vi "WPI_CameraPublish Settings.vi"(8 "Name":string, 9 "Table":string, 11 "CameraDevRef":T1) -> ()   [LabVIEW 2017]
uses:
  <vilib>/Rock Robotics/WPI/Camera/WPI_CameraDevRef.ctl
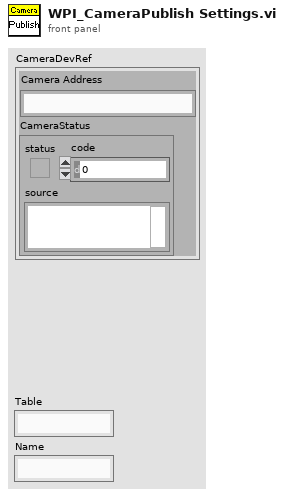
[diagram p1: front panel]
types:
  T1 = typedef "WPI_CameraDevRef.ctl" = cluster{"Camera Address":string, "CameraStatus":errorcluster}
  T2 = typedef "WPI_CameraImageSize.ctl" = enum16{"640x480", "320x240", "160x120", "Custom"}
  T3 = typedef "WPI_CameraFrameRate.ctl" = u32
  T4 = typedef "WPI_CameraExposure Values.ctl" = enum16{"Auto", "Flicker-free 50 Hz", "Flicker-free 60 Hz", "Hold current", "Custom"}
  T5 = typedef "WPI_CameraWhite Balance Values.ctl" = enum16{"Auto", "Fixed indoor", "Fixed outdoor 1", "Fixed outdoor 2", "Fixed fluorescent 1", "Fixed fluorescent 2", "Hold current", "Custom"}
  T6 = typedef "WPI_CameraExposure Priority Values.ctl" = enum16{"None", "Prioritize frame rate", "Prioritize image quality"}
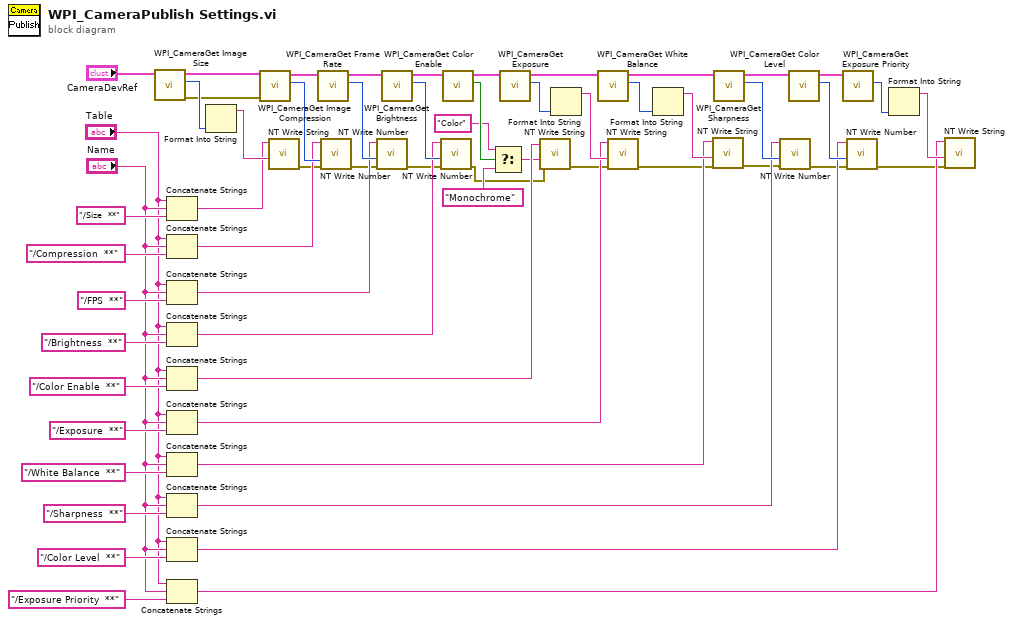
[diagram p0: block diagram]
diagram:
  n1 = call <vilib>:"WPI_CameraGet Image Size.vi"("CameraDevRef"="CameraDevRef") -> ("error out"=w10:errorcluster, "Image Size"=w58:T2, "CameraDevRef Out"=w54:T1)  [unwired: 7 in, 1 out]
  n2 = Concatenate Strings("Table", "Name", "/Size  **") -> (w49:string)
  n3 = Concatenate Strings("Table", "Name", "/Compression  **") -> (w48:string)
  n4 = Concatenate Strings("Table", "Name", "/FPS  **") -> (w47:string)
  n5 = Concatenate Strings("Table", "Name", "/Brightness  **") -> (w43:string)
  n6 = Concatenate Strings("Table", "Name", "/Color Enable  **") -> (w15:string)
  n7 = Concatenate Strings("Table", "Name", "/Exposure  **") -> (w32:string)
  n8 = Concatenate Strings("Table", "Name", "/White Balance  **") -> (w31:string)
  n9 = Concatenate Strings("Table", "Name", "/Sharpness  **") -> (w19:string)
  n10 = Concatenate Strings("Table", "Name", "/Color Level  **") -> (w18:string)
  n11 = Concatenate Strings("Table", "Name", "/Exposure Priority  **") -> (w17:string)
  n12 = Format Into String(w58) -> (resulting string=w59:string)  [unwired: 3 in, 1 out]
  n13 = call <vilib>:"WPI_CameraGet Image Compression.vi"("error in (no error)"=w10, "CameraDevRef"=w54) -> ("Compression"=w55:i32, "CameraDevRef Out"=w57:T1)  [unwired: 7 in, 1 out]
  n14 = call <vilib>:"NT Write String.vi"("String"=w59, "Name"=w49) -> ("error out"=w9:errorcluster)  [unwired: 9 in]
  n15 = call <vilib>:"WPI_CameraGet Frame Rate.vi"("CameraDevRef"=w57) -> ("Frame Rate (fps)"=w56:T3, "CameraDevRef Out"=w46:T1)  [unwired: 8 in, 1 out]
  n16 = call <vilib>:"NT Write Number.vi"("error in"=w9, "Numeric"=w55, "Name"=w48) -> ("error out"=w8:errorcluster)  [unwired: 8 in]
  n17 = call <vilib>:"NT Write Number.vi"("error in"=w8, "Numeric"=w56, "Name"=w47) -> ("error out"=w7:errorcluster)  [unwired: 8 in]
  n18 = call <vilib>:"WPI_CameraGet Brightness.vi"("CameraDevRef"=w46) -> ("Brightness"=w45:i32, "CameraDevRef Out"=w42:T1)  [unwired: 8 in, 1 out]
  n19 = call <vilib>:"NT Write Number.vi"("error in"=w7, "Numeric"=w45, "Name"=w43) -> ("error out"=w6:errorcluster)  [unwired: 8 in]
  n20 = call <vilib>:"WPI_CameraGet Color Enable.vi"("CameraDevRef"=w42) -> ("Color Enabled"=w13:bool, "CameraDevRef Out"=w41:T1)  [unwired: 8 in, 1 out]
  n21 = Select(t="Color", s=w13, f="Monochrome") -> (s? t:f=w14:string)
  n22 = call <vilib>:"WPI_CameraGet Exposure.vi"("CameraDevRef"=w41) -> ("Exposure"=w37:T4, "CameraDevRef Out"=w40:T1)  [unwired: 7 in, 2 out]
  n23 = call <vilib>:"NT Write String.vi"("error in"=w6, "String"=w14, "Name"=w15) -> ("error out"=w5:errorcluster)  [unwired: 8 in]
  n24 = Format Into String(w37) -> (resulting string=w36:string)  [unwired: 3 in, 1 out]
  n25 = call <vilib>:"WPI_CameraGet White Balance.vi"("CameraDevRef"=w40) -> ("White Balance"=w39:T5, "CameraDevRef Out"=w30:T1)  [unwired: 7 in, 2 out]
  n26 = call <vilib>:"NT Write String.vi"("error in"=w5, "String"=w36, "Name"=w32) -> ("error out"=w4:errorcluster)  [unwired: 8 in]
  n27 = Format Into String(w39) -> (resulting string=w38:string)  [unwired: 3 in, 1 out]
  n28 = call <vilib>:"NT Write String.vi"("error in"=w4, "String"=w38, "Name"=w31) -> ("error out"=w3:errorcluster)  [unwired: 8 in]
  n29 = call <vilib>:"WPI_CameraGet Sharpness.vi"("CameraDevRef"=w30) -> ("Sharpness"=w27:i32, "CameraDevRef Out"=w29:T1)  [unwired: 8 in, 1 out]
  n30 = call <vilib>:"NT Write Number.vi"("error in"=w3, "Numeric"=w27, "Name"=w19) -> ("error out"=w2:errorcluster)  [unwired: 8 in]
  n31 = call <vilib>:"WPI_CameraGet Color Level.vi"("CameraDevRef"=w29) -> ("Color Level"=w26:i32, "CameraDevRef Out"=w28:T1)  [unwired: 8 in, 1 out]
  n32 = call <vilib>:"WPI_CameraGet Exposure Priority.vi"("CameraDevRef"=w28) -> ("Exposure Priority"=w25:T6)  [unwired: 8 in, 2 out]
  n33 = call <vilib>:"NT Write Number.vi"("error in"=w2, "Numeric"=w26, "Name"=w18) -> ("error out"=w1:errorcluster)  [unwired: 8 in]
  n34 = Format Into String(w25) -> (resulting string=w24:string)  [unwired: 3 in, 1 out]
  n35 = call <vilib>:"NT Write String.vi"("error in"=w1, "String"=w24, "Name"=w17) -> ()  [unwired: 8 in, 1 out]
